vi "WritePort.vi"(8 "error in (no error)":errorcluster, 11 "Port":string[](array[string])) -> (0 "error out":errorcluster)   [LabVIEW 2013]
uses:
  SourceCode/GlobalValue.vi
  <vilib>/Utility/config.llb/Write Key (String).vi
  <vilib>/Utility/config.llb/NI_LVConfig.lvlib
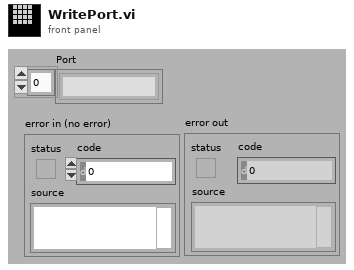
[diagram p1: front panel]
types:
  T1 = typedef "NI_LVConfig.lvlib/Config Data RefNum.ctl" = refnum<k1>
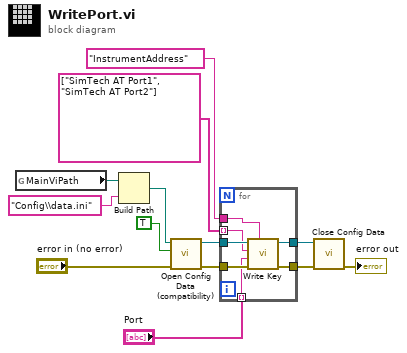
[diagram p0: block diagram]
diagram:
  n1 = global read "GlobalValue.vi" "MainViPath"() -> (w4:path)
  n2 = Build Path(base path=w4, name or relative path="Config\\data.ini" ("名称或相对路径")) -> (appended path=w5:path)
  n3 = call <vilib>:"Open Config Data (compatibility).vi"("error in (no error)"="error in (no error)", "create file if necessary (T)"=TRUE, "configuration file path"=w5) -> ("error out"=w11:errorcluster, "refnum"=w12:T1)  [unwired: 6 in, 1 out]
  n4 = for {
    tunnel: w12 -> [w20]
    tunnel: w11 -> [w19]
    tunnel: [w18] -> w9
    tunnel: [w17] -> w10
    tunnel: "InstrumentAddress" ("ModelName") -> [w16]
    tunnel: string[] ["SimTech AT Port1", "SimTech AT Port2"] -> [w15] mode=indexing
    tunnel: "Port" -> [w14] mode=indexing
    n5 = call-poly <vilib>:"Write Key.vi"("section"=w16, "error in (no error)"=w19, "value"=w14, "key"=w15, "refnum"=w20) -> ("error out"=w18:errorcluster, "refnum out"=w17:T1)  [unwired: 4 in, 1 out]
  }
  n6 = call <vilib>:"Close Config Data.vi"("error in (no error)"=w9, "refnum"=w10) -> ("error out"=→"error out":errorcluster)  [unwired: 1 in, 8 out]
